vi "Register for Events (Multiple PyObjects by Enum).vi"(8 "error in (no error)":errorcluster, 9 "Variant":variant, 11 "JKI_Python_Server in":refnum<class "Server.lvclass">) -> (0 "error out":errorcluster, 1 "Python":T1, 3 "JKI_Python_Server out":refnum<class "Server.lvclass">)   [LabVIEW 2013, in "JKI_Python_Bridge_for_LV.lvlib" / "Server.lvclass"]
uses:
  Server.lvclass
  Type Definitions/Python Method Call - Event Registration.ctl
  Call/Call.lvclass
  Type Definitions/Public Events - Cluster.ctl
  <userlib>/_OpenG.lib/lvdata/lvdata.llb/Get TDEnum from Data__ogtk.vi
  <userlib>/_OpenG.lib/array/array.llb/Conditional Auto-Indexing Tunnel__ogtk.vi
  <userlib>/_OpenG.lib/array/array.llb/Conditional Auto-Indexing Tunnel (String)__ogtk.vi
  <userlib>/_OpenG.lib/array/array.llb/Remove Duplicates from 1D Array__ogtk.vi
  <userlib>/_OpenG.lib/array/array.llb/Remove Duplicates from 1D Array (String)__ogtk.vi
  <userlib>/_OpenG.lib/error/error.llb/Build Error Cluster__ogtk.vi
  <userlib>/_OpenG.lib/lvdata/lvdata.llb/Get Strings from Enum__ogtk.vi
  <userlib>/_OpenG.lib/array/array.llb/Search Array__ogtk.vi
  <userlib>/_OpenG.lib/array/array.llb/Search 1D Array (String)__ogtk.vi
  <userlib>/_OpenG.lib/array/array.llb/Index Array Elements__ogtk.vi
  <userlib>/_OpenG.lib/array/array.llb/Index 1D Array Elements (String)__ogtk.vi
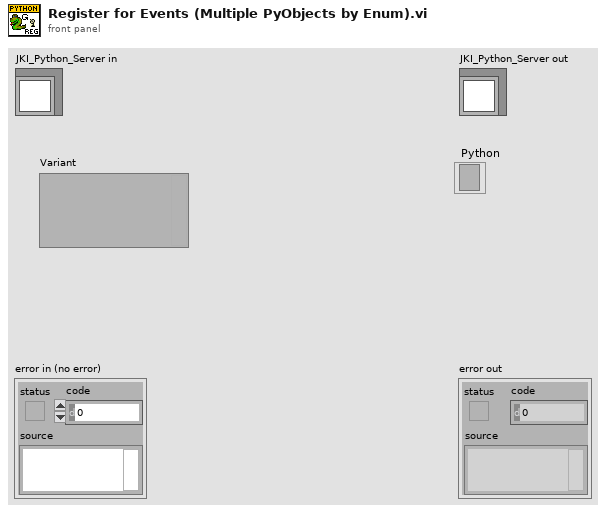
[diagram p1: front panel]
types:
  T1 = typedef "JKI_Python_Bridge_for_LV.lvlib/Server.lvclass/Python Method Call - Event Registration.ctl" = refnum<event-registration>
  T2 = typedef "JKI_Python_Bridge_for_LV.lvlib/Server.lvclass/Python Object and Method Names - Cluster.ctl" = cluster{"PyObject Name":string, "Functions":T3[]}
  T3 = typedef "JKI_Python_Bridge_for_LV.lvlib/Server.lvclass/Python Method.ctl" = cluster{"Name":string, "Arguments":string[], "Documentation":string}
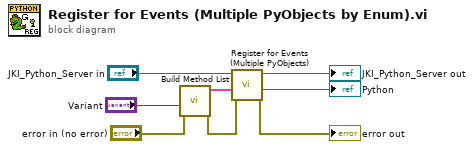
[diagram p0: block diagram]
diagram:
  n1 = call "Build Method List.vi"("error in (no error)"="error in (no error)", "Method List (VEnum)"="Variant") -> ("error out"=w1:errorcluster, "PyObjects"=w3:T2[])  [unwired: 8 in]
  n2 = call "Register for Events (Multiple PyObjects).vi"("error in (no error)"=w1, "PyObjects"=w3, "JKI_Python_Server in"="JKI_Python_Server in") -> ("error out"=→"error out":errorcluster, "Python"=→"Python":T1, "JKI_Python_Server out"=→"JKI_Python_Server out":refnum<class "Server.lvclass">)  [unwired: 6 in]
